vi "laserGetPower.vi"(8 "error in (no error)":errorcluster, 10 "ms to wait (5)":u32=5, 11 "VISA resource name":refnum<visa-resource-name>) -> (0 "error out":errorcluster, 2 "Power, mW":dbl, 3 "VISA resource name out":refnum<visa-resource-name>)   [LabVIEW 2011]
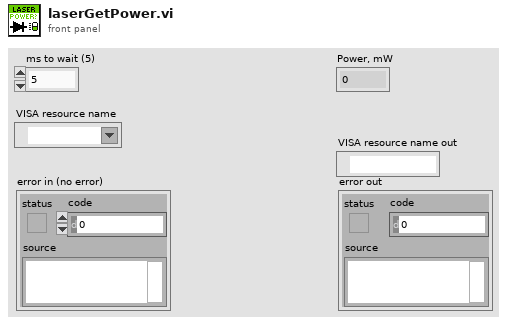
[diagram p1: front panel]
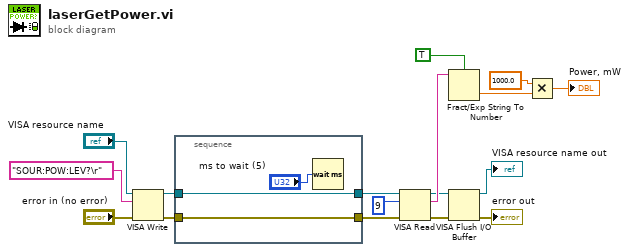
[diagram p0: block diagram]
diagram:
  n1 = VISA Write(VISA resource name="VISA resource name", write buffer="SOUR:POW:LEV?\r", error in (no error)="error in (no error)") -> (VISA resource name out=w16:refnum<visa-resource-name>, error out=w15:errorcluster)  [unwired: 1 out]
  n2 = stacked-sequence {
    tunnel: w16 -> [w20]
    tunnel: [w20] -> w14
    tunnel: [w19] -> w13
    tunnel: w15 -> [w19]
    frame #0 {
      n3 = Wait (ms)(milliseconds to wait="ms to wait (5)") -> ()  [unwired: 1 out]
    }
  }
  n4 = VISA Read(VISA resource name=w14, byte count=u32 9, error in (no error)=w13) -> (VISA resource name out=w8:refnum<visa-resource-name>, read buffer=w11:string, error out=w7:errorcluster)  [unwired: 1 out]
  n5 = Fract/Exp String To Number(use system decimal point (T)=TRUE, string=w11) -> (number=w3:dbl)  [unwired: 2 in, 1 out]
  n6 = VISA Flush I/O Buffer(VISA resource name=w8, error in (no error)=w7) -> (VISA resource name out=→"VISA resource name out":refnum<visa-resource-name>, error out=→"error out":errorcluster)  [unwired: 1 in]
  n7 = Multiply(x=1000.0, y=w3) -> (x*y=→"Power, mW":dbl)
